vi "Get desired piece.vi"(11 "type":enum16{"Z", "I", "O", "S", "L", "J", "T", "N"}(ring)) -> ()   [LabVIEW 2018]
uses:
  vision/vision info 2.vi
panel:
  out "needed":bool
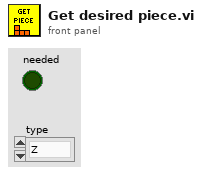
[diagram p1: front panel]
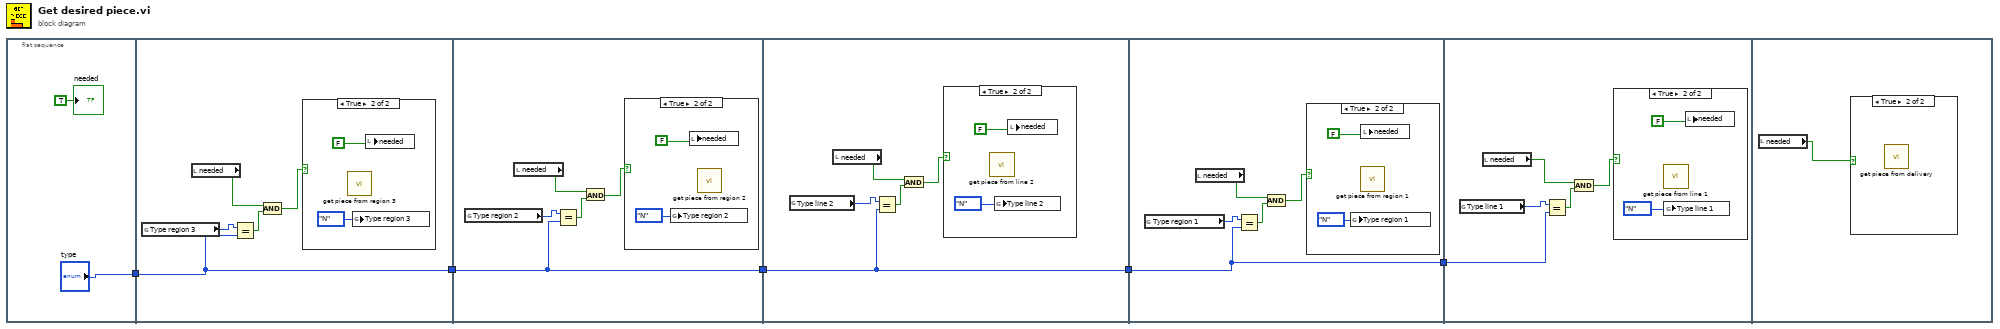
[diagram p0: block diagram]
diagram:
  n1 = flat-sequence {
    tunnel: ["type"] -> w5
    tunnel: w5 -> [w8]
    tunnel: [w8] -> w4
    tunnel: w4 -> [w15]
    tunnel: [w15] -> w3
    tunnel: w3 -> [w22]
    tunnel: [w22] -> w2
    tunnel: w2 -> [w29]
    tunnel: [w29] -> w1
    tunnel: w1 -> [w36]
    frame #0 {
      "needed" <- TRUE ("taken")
    }
    frame #1 {
      n2 = global read "vision info 2.vi" "Type region 3"() -> (w12:enum16{"Z", "I", "O", "S", "L", "J", "T", "N"})
      n3 = local read "needed"() -> (w10:bool)
      n4 = Equal?(x=w12, y=w8) -> (x = y?=w11:bool)
      n5 = And(x=w10, y=w11) -> (x .and. y?=w9:bool)
      n6 = case shown="True" w9 {
        frame False {
        }
        frame True {
          n7 = call "get piece from region 3.vi"() -> ()  [unwired: 12 in]
          n8 = global write "vision info 2.vi" "Type region 3"(enum16{"Z", "I", "O", "S", "L", "J", "T", "N"}."N" ("Type region 3")) -> ()
          n9 = local write "needed"(FALSE ("taken")) -> ()
        }
      }
    }
    frame #2 {
      n10 = global read "vision info 2.vi" "Type region 2"() -> (w19:enum16{"Z", "I", "O", "S", "L", "J", "T", "N"})
      n11 = local read "needed"() -> (w17:bool)
      n12 = Equal?(x=w19, y=w15) -> (x = y?=w18:bool)
      n13 = And(x=w17, y=w18) -> (x .and. y?=w16:bool)
      n14 = case shown="True" w16 {
        frame False {
        }
        frame True {
          n15 = global write "vision info 2.vi" "Type region 2"(enum16{"Z", "I", "O", "S", "L", "J", "T", "N"}."N" ("Type region 3")) -> ()
          n16 = local write "needed"(FALSE ("taken")) -> ()
          n17 = call "get piece from region 2.vi"() -> ()  [unwired: 12 in]
        }
      }
    }
    frame #3 {
      n18 = global read "vision info 2.vi" "Type line 2"() -> (w26:enum16{"Z", "I", "O", "S", "L", "J", "T", "N"})
      n19 = local read "needed"() -> (w24:bool)
      n20 = Equal?(x=w26, y=w22) -> (x = y?=w25:bool)
      n21 = And(x=w24, y=w25) -> (x .and. y?=w23:bool)
      n22 = case shown="True" w23 {
        frame False {
        }
        frame True {
          n23 = call "get piece from line 2.vi"() -> ()  [unwired: 12 in]
          n24 = global write "vision info 2.vi" "Type line 2"(enum16{"Z", "I", "O", "S", "L", "J", "T", "N"}."N" ("Type region 3")) -> ()
          n25 = local write "needed"(FALSE ("taken")) -> ()
        }
      }
    }
    frame #4 {
      n26 = global read "vision info 2.vi" "Type region 1"() -> (w33:enum16{"Z", "I", "O", "S", "L", "J", "T", "N"})
      n27 = local read "needed"() -> (w31:bool)
      n28 = Equal?(x=w33, y=w29) -> (x = y?=w32:bool)
      n29 = And(x=w31, y=w32) -> (x .and. y?=w30:bool)
      n30 = case shown="True" w30 {
        frame False {
        }
        frame True {
          n31 = global write "vision info 2.vi" "Type region 1"(enum16{"Z", "I", "O", "S", "L", "J", "T", "N"}."N" ("Type region 3")) -> ()
          n32 = call "get piece from region 1.vi"() -> ()  [unwired: 12 in]
          n33 = local write "needed"(FALSE ("taken")) -> ()
        }
      }
    }
    frame #5 {
      n34 = global read "vision info 2.vi" "Type line 1"() -> (w40:enum16{"Z", "I", "O", "S", "L", "J", "T", "N"})
      n35 = local read "needed"() -> (w38:bool)
      n36 = Equal?(x=w40, y=w36) -> (x = y?=w39:bool)
      n37 = And(x=w38, y=w39) -> (x .and. y?=w37:bool)
      n38 = case shown="True" w37 {
        frame False {
        }
        frame True {
          n39 = call "get piece from line 1.vi"() -> ()  [unwired: 12 in]
          n40 = global write "vision info 2.vi" "Type line 1"(enum16{"Z", "I", "O", "S", "L", "J", "T", "N"}."N" ("Type region 3")) -> ()
          n41 = local write "needed"(FALSE ("taken")) -> ()
        }
      }
    }
    frame #6 {
      n42 = local read "needed"() -> (w43:bool)
      n43 = case shown="True" w43 {
        frame False {
        }
        frame True {
          n44 = call "get piece from delivery.vi"() -> ()  [unwired: 12 in]
        }
      }
    }
  }
